vi "ARRAY TO NUMBER.vi"() -> ()   [LabVIEW 2019]
panel:
  out "number":u32
  in  "Array":bool[](array[boolean])
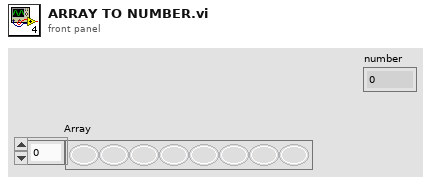
[diagram p1: front panel]
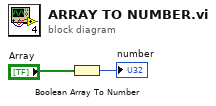
[diagram p0: block diagram]
diagram:
  n1 = Boolean Array To Number(Boolean array="Array") -> (number=→"number":u32)
